vi "BuildZLUT.vi"(11 "MeasureConfig":T2={"Bead locations"=[{"X"=0, "Y"=0}], "ROI"=200, "Experiment base path"=path "", "Image output subdir"="images", "Output mode"=enum."None", "Traces output subdir"="traces", "QTrk Settings"={"Image width"=150, "Image height"=150, "Number of threads (CPU based)"=-1, "CUDA Device"=-2, "COM Background correction factor"=0.0, "ZLUT MinRadius"=8.0, "ZLUT Radial sample density"=5.0, "ZLUT Angular sample density"=2.0, "ZLUT ROI Coverage"=0.7, "QI Iterations"=1, "QI MinRadius"=2.0, "QI Radial sample density"=5.0, "QI Angular sample density"=2.0, "QI ROI Coverage"=0.7, "QI Angular Step \nIteration Factor"=0.8, "XCOR Profile Length"=1, "XCOR Profile Width"=128, "XCOR Iterations"=32, "Gaussian 2D Fit Iterations"=2, "Gaussian 2D Sigma (pixels)"=3.0, "Downsample"=0}, "Tracking Config"={"Number of steps"=0, "ZLUT stepsize (um)"=0.0, "Z correction factor"=0.0, "Start piezo Z (um)"=0.0, "Pixel size (nm)"=0.0, "2D Localization Type"=enum."Quadrant Interpolation", "Z Command (None)"=enum."Nothing", "Z Piezo scale"=FALSE}, "Experiment Name"="", "Program"={"Commands"=[], "Motor Axis accuracy conditions"={"Magnet Z"=0.0, "Magnet rotation"=0.0, "Camera"={"X"=0.0, "Y"=0.0}, "Piezo XY"={"X"=0.0, "Y"=0.0}, "Piezo Z"=0.0}, "Axis flags"={"Magnet Z"=FALSE, "Magnet rotation"=FALSE, "Camera"={"X"=FALSE, "Y"=FALSE}, "Piezo XY"={"X"=FALSE, "Y"=FALSE}, "Piezo Z"=FALSE}}, "ZLUT"=[], "Camera settings"={"Framerate (Hz)"=60, "Exposure time (us)"=5000, "Image size"={"Width"=1280, "Height"=1024}, "Number of buffers"=30}, "Experiment Script"="", "Max frames in memory"=10000, "Save traces as binary"=FALSE, "Pixel Calibration Gain Image"="camera_calib_gain.bin", "Pixel Calibration Offset Image"="camera_calib_offset.bin", "Use pixel calibration images"=FALSE, "Internal camera settings"="", "Trace write interval"=100} {"QTrk Settings"."QI ROI Coverage" format="%_2g"; "QTrk Settings"."QI MinRadius" format="%.2f"; "QTrk Settings"."QI Angular sample density" format="%.3f"; "QTrk Settings"."QI Radial sample density" format="%.2f"; "QTrk Settings"."ZLUT Radial sample density" format="%.2f"; "QTrk Settings"."ZLUT MinRadius" format="%.2f"}) -> (2 "Is cancelled?":bool, 3 "ZLUT":sgl[][][](array[numeric]))   [LabVIEW 2011]
uses:
  Typedefs/MeasureConfigType.ctl
  Typedefs/MeasureConfigOutputMode.ctl
  qtrk/QTrkLVBinding/QTrkSettings.ctl
  Typedefs/TrackingConfigType.ctl
  qtrk/QTrkLVBinding/QTrkLocalizationType.ctl
  qtrk/QTrkLVBinding/QTrkZCommandType.ctl
  ExperimentProgram/ExperimentProgramType.ctl
  ExperimentProgram/ExProgCommandType.ctl
  ExperimentProgram/ExProgCommandEnumType.ctl
  Motors/MotorAxisEnum.ctl
  Motors/MotorPosType.ctl
  Typedefs/XYf.ctl
  Motors/MotorPosFlagsType.ctl
  Camera/GenericCameraConfigType.ctl
  <vilib>/vision/Image Controls.llb/IMAQ Image.ctl
  Camera/CIGrabControlMsg.ctl
  Camera/CIGrabControlMsgEnum.ctl
  GlobalVariables.vi
panel:
  in  "Wait frames after motor move":i32=1
  in  "thread id":i32
  in  "Get debug image?":bool
  out "dbg image":sgl[][](graph)
  in  "Grab Framerate (Hz)":i32=20
  out "Image":T1(plugin-control)
  in  "Check for motor position?":bool=TRUE
  in  "Image available?":bool
  in  "stop capturing":bool
  out "total result count":i32
  out "QTrk result count":i32
  out "Piezo Z":sgl
  in  "Cancel":bool
  out "Frame #":i32
  out "last image grabbed":T1
  out "Total # of steps":i32
  out "Step":i32
  # "Building Z lookup table..."
  # "(used for commands with string parameters)"
  # "-2: Use all devices\n-1: Use best device"
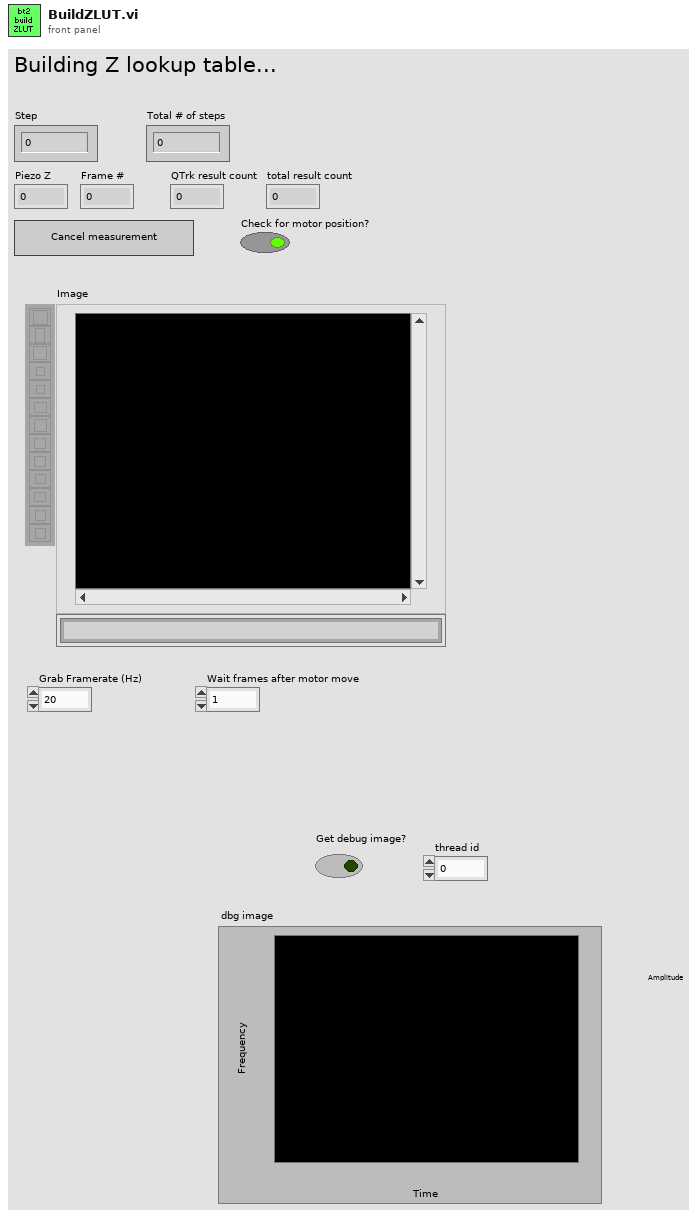
[diagram p1: front panel]
types:
  T1 = typedef "IMAQ Image.ctl" = refnum<image>
  T2 = typedef "MeasureConfigType.ctl" = cluster{"Bead locations":cluster{"X":i32, "Y":i32}[], "ROI":i32, "Experiment base path":path, "Image output subdir":string, "Output mode":T3, "Traces output subdir":string, "QTrk Settings":T4, "Tracking Config":T5, "Experiment Name":string, "Program":T8, "ZLUT":sgl[][][], "Camera settings":T15, "Experiment Script":string, "Max frames in memory":i32, "Save traces as binary":bool, "Pixel Calibration Gain Image":string, "Pixel Calibration Offset Image":string, "Use pixel calibration images":bool, "Internal camera settings":string, "Trace write interval":i32}
  T3 = typedef "MeasureConfigOutputMode.ctl" = enum16{"None", "Track", "SaveImages"}
  T4 = typedef "QTrkSettings.ctl" = cluster{"Image width":i32, "Image height":i32, "Number of threads (CPU based)":i32, "CUDA Device":i32, "COM Background correction factor":sgl, "ZLUT MinRadius":sgl, "ZLUT Radial sample density":sgl, "ZLUT Angular sample density":sgl, "ZLUT ROI Coverage":sgl, "QI Iterations":i32, "QI MinRadius":sgl, "QI Radial sample density":sgl, "QI Angular sample density":sgl, "QI ROI Coverage":sgl, "QI Angular Step \nIteration Factor":sgl, "XCOR Profile Length":i32, "XCOR Profile Width":i32, "XCOR Iterations":i32, "Gaussian 2D Fit Iterations":i32, "Gaussian 2D Sigma (pixels)":sgl, "Downsample":i32}
  T5 = typedef "TrackingConfigType.ctl" = cluster{"Number of steps":i32, "ZLUT stepsize (um)":sgl, "Z correction factor":sgl, "Start piezo Z (um)":sgl, "Pixel size (nm)":sgl, "2D Localization Type":T6, "Z Command (None)":T7, "Z Piezo scale":bool}
  T6 = typedef "QTrkLocalizationType.ctl" = enum16{"Center-of-Mass", "1D Cross-Correlation", "Quadrant Interpolation", "Gaussian 2D MLE", "QI + ZLUTAlign", "ZLUTAlign", "QI + FourierLUT"}
  T7 = typedef "QTrkZCommandType.ctl" = enum16{"Nothing", "ComputeZ", "BuildRadialZLUT", "BuildImageZLUT", "RadialZLUT+ImageZLUT"}
  T8 = typedef "ExperimentProgramType.ctl" = cluster{"Commands":T9[], "Motor Axis accuracy conditions":T12, "Axis flags":T14}
  T9 = typedef "ExProgCommandType.ctl" = cluster{"cmd":T10, "axis":T11, "value/pos":dbl, "speed":dbl, "name":string}
  T10 = typedef "ExProgCommandEnumType.ctl" = enum16{"wait", "move", "acquire", "idle", "rmove", "when", "section", "stop"}
  T11 = typedef "MotorAxisEnum.ctl" = enum16{"no axis", "magrot", "magpos", "px", "py", "pz", "camx", "camy"}
  T12 = typedef "MotorPosType.ctl" = cluster{"Magnet Z":dbl, "Magnet rotation":dbl, "Camera":T13, "Piezo XY":T13, "Piezo Z":dbl}
  T13 = typedef "XYf.ctl" = cluster{"X":sgl, "Y":sgl}
  T14 = typedef "MotorPosFlagsType.ctl" = cluster{"Magnet Z":bool, "Magnet rotation":bool, "Camera":cluster{"X":bool, "Y":bool}, "Piezo XY":cluster{"X":bool, "Y":bool}, "Piezo Z":bool}
  T15 = typedef "GenericCameraConfigType.ctl" = cluster{"Framerate (Hz)":i32, "Exposure time (us)":i32, "Image size":cluster{"Width":i32, "Height":i32}, "Number of buffers":i32}
  T16 = typedef "MotorStateType.ctl" = cluster{"Enabled?":bool, "Current Position":T12, "Update counter":i32}
  T17 = typedef "QTrkInstance.ctl" = cluster{"QTrk Pointer":u64}
  T18 = typedef "QTrkComputedSettings.ctl" = cluster{"QTrk Settings":T4, "Derived settings":cluster{"ZLUT Radial Steps":i32, "ZLUT Angular Steps":i32, "ZLUT Max Radius":sgl, "QI Radial Steps":i32, "QI Angular Steps\nPer Quadrant":i32, "QI Max Radius":sgl}}
  T19 = typedef "CIGrabType.ctl" = refnum<vi>
  T20 = typedef "CmdData_NewFrame.ctl" = cluster{"Buffer Image":T1, "Frame #":i32, "Hardware ROI Index":i32, "Timestamp":dbl, "Type":T21}
  T21 = typedef "CmdEnum_CameraFrameType.ctl" = enum16{"Full", "HardwareROI", "EndGrabMarker"}
  T22 = typedef "CIGrabControlMsg.ctl" = cluster{"Msg":T23}
  T23 = typedef "CIGrabControlMsgEnum.ctl" = enum16{"Stop", "EnableTracking", "DisableTracking"}
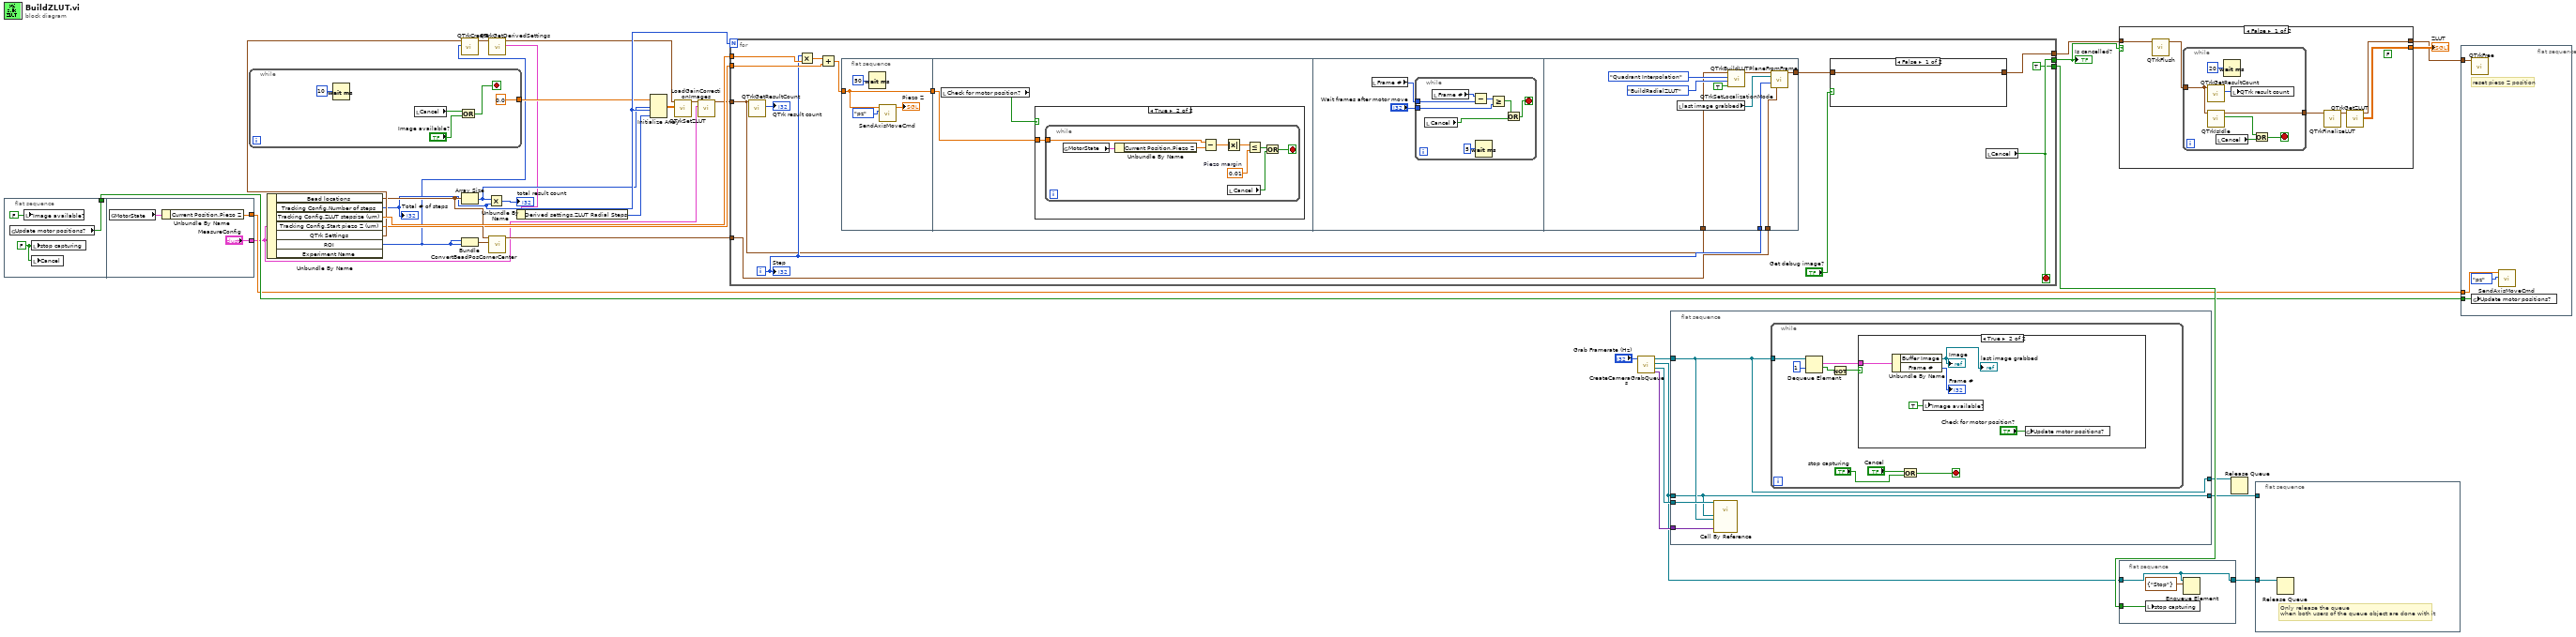
[diagram p0: block diagram]
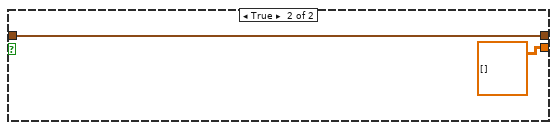
[diagram p3: hidden frame]
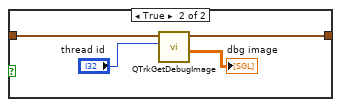
[diagram p4: hidden frame]
diagram:
  n1 = flat-sequence {
    tunnel: [w35] -> w17
    tunnel: ["MeasureConfig"] -> w12
    tunnel: [w38] -> w16
    frame #0 {
      w36 = FALSE ("Cancel")
      n2 = global read "GlobalVariables.vi" "Update motor positions?"() -> (w35:bool)
      n3 = local write "Image available?"(FALSE ("Image available?")) -> ()
      n4 = local write "stop capturing"(w36) -> ()
      n5 = local write "Cancel"(w36) -> ()
    }
    frame #1 {
      n6 = global read "GlobalVariables.vi" "MotorState"() -> (w39:T16)
      n7 = Unbundle By Name(w39) -> ("Current Position.Piezo Z"=w38:dbl)
    }
  }
  n8 = while {
    tunnel: [sgl 0.0 ("element")] -> w22
    stop <- w41 stop-if-true
    n9 = Wait (ms)(milliseconds to wait=u32 10) -> ()  [unwired: 1 out]
    n10 = local read "Cancel"() -> (w43:bool)
    n11 = Or(x=w43, y="Image available?") -> (x .or. y?=w41:bool)
  }
  n12 = Unbundle By Name(w12) -> ("Bead locations"=w31:cluster{"X":i32, "Y":i32}[], "Tracking Config.Number of steps"=w25:i32, "Tracking Config.ZLUT stepsize (um)"=w34:sgl, "Tracking Config.Start piezo Z (um)"=w21:sgl, "QTrk Settings"=w33:T4, "ROI"=w19:i32)  [unwired: 1 out]
  "Total # of steps" <- w25
  n13 = call "QTrkCreate.vi"("ROI"=w19, "QTrk Settings"=w33) -> ("QTrk Instance"=w15:T17)  [unwired: 3 in, 2 out]
  n14 = Array Size(array=w31) -> (size(s)=w20:i32)
  n15 = Bundle("ROI"=w19, "ROI"=w19) -> (w18:cluster{"ROI":i32, "ROI":i32})  [unwired: 1 in]
  n16 = Multiply(x=w20, y=w25) -> (x*y=→"total result count":i32)
  n17 = call "QTrkGetDerivedSettings.vi"("QTrk Instance"=w15) -> ("Derived settings"=w14:T18, "QTrk Instance (out)"=w1:T17)  [unwired: 5 in, 4 out]
  n18 = call "ConvertBeadPosCornerCenter.vi"("ROI Size"=w18, "Center-based bead locations"=w31) -> ("Corner-based bead pos (out)"=w30:cluster{"X":i32, "Y":i32}[])  [unwired: 8 in, 1 out]
  n19 = Unbundle By Name(w14) -> ("Derived settings.ZLUT Radial Steps"=w13:i32)
  n20 = Initialize Array(w22, w20, w25, w13) -> (w32:sgl[][][])
  n21 = call "QTrkSetZLUT.vi"("ZLUT"=w32, "QTrk Instance"=w1) -> ("QTrk Instance"=w11:T17)  [unwired: 8 in, 1 out]
  n22 = call "LoadGainCorrectionImages.vi"("MeasureConfig"=w12, "QTrk Instance in"=w11) -> ("QTrk Instance out"=w10:T17)  [unwired: 9 in]
  n23 = for {
    N: w25 -> [_]
    tunnel: w34 -> [w59]
    tunnel: w21 -> [w57]
    tunnel: w10 -> [w52]
    tunnel: [w46] -> w27
    tunnel: w30 -> [w54]
    tunnel: [w53] -> w26
    tunnel: [TRUE ("stop capturing")] -> w23
    i -> [w55]
    stop <- w53 stop-if-true
    n24 = call "QTrkGetResultCount.vi"("QTrk Instance"=w52) -> ("result count"=→"QTrk result count":i32)  [unwired: 4 in, 2 out]
    n25 = Multiply(x=w55, y=w59) -> (x*y=w58:sgl)
    n26 = Add(x=w58, y=w57) -> (x+y=w56:sgl)
    n27 = flat-sequence {
      tunnel: w56 -> [w67]
      tunnel: [w67] -> w49
      tunnel: w49 -> [w70]
      tunnel: w52 -> [w96]
      tunnel: w55 -> [w94]
      tunnel: [w92] -> w47
      tunnel: w54 -> [w93]
      frame #0 {
        n28 = Wait (ms)(milliseconds to wait=u32 50) -> ()  [unwired: 1 out]
        n29 = call "SendAxisMoveCmd.vi"("axis"=MotorAxisEnum."pz", "Position"=w67) -> ("Limited pos"=→"Piezo Z":dbl)  [unwired: 9 in]
      }
      frame #1 {
        n30 = local read "Check for motor position?"() -> (w69:bool)
        n31 = case shown="True" w69 {
          tunnel: w70 -> [_ w71]
          frame False {
          }
          frame True {
            n32 = while {
              tunnel: w71 -> [w77]
              stop <- w78 stop-if-true
              w73 = 0.01  # Piezo margin
              n33 = global read "GlobalVariables.vi" "MotorState"() -> (w80:T16)
              n34 = Unbundle By Name(w80) -> ("Current Position.Piezo Z"=w76:dbl)
              n35 = Subtract(x=w77, y=w76) -> (x-y=w75:dbl)
              n36 = Absolute Value(x=w75) -> (abs(x)=w74:dbl)
              n37 = local read "Cancel"() -> (w79:bool)
              n38 = Less Or Equal?(x=w74, y=w73) -> (x <= y?=w72:bool)
              n39 = Or(x=w72, y=w79) -> (x .or. y?=w78:bool)
            }
          }
        }
      }
      frame #2 {
        n40 = local read "Frame #"() -> (w82:i32)
        n41 = while {
          tunnel: w82 -> [w89]
          tunnel: "Wait frames after motor move" -> [w87]
          stop <- w84 stop-if-true
          n42 = local read "Cancel"() -> (w83:bool)
          n43 = local read "Frame #"() -> (w90:i32)
          n44 = Subtract(x=w90, y=w89) -> (x-y=w88:i32)
          n45 = Wait (ms)(milliseconds to wait=u32 5) -> ()  [unwired: 1 out]
          n46 = Greater Or Equal?(x=w88, y=w87) -> (x >= y?=w85:bool)
          n47 = Or(x=w85, y=w83) -> (x .or. y?=w84:bool)
        }
      }
      frame #3 {
        n48 = local read "last image grabbed"() -> (w91:T1)
        n49 = call "QTrkSetLocalizationMode.vi"("Normalize profile"=TRUE, "Z Command"=QTrkZCommandType."BuildRadialZLUT", "2D Localization Type"=QTrkLocalizationType."Quadrant Interpolation", "QTrk Instance"=w96) -> ("QTrk Instance"=w95:T17)  [unwired: 7 in]
        n50 = call "QTrkBuildLUTPlaneFromFrame.vi"("QTrk Instance"=w95, "Image"=w91, "plane"=w94, "ROI Positions (corner-based)"=w93) -> ("QTrk Instance"=w92:T17)  [unwired: 11 in]
      }
    }
    n51 = case shown="False" "Get debug image?" {
      tunnel: w47 -> [w60 w64]
      tunnel: [w60 w63] -> w46
      frame False {
      }
      frame True {
        n52 = call "QTrkGetDebugImage.vi"("id"="thread id", "QTrk Instance"=w64) -> ("data"=→"dbg image":sgl[][], "QTrk Instance (out)"=w63:T17)  [unwired: 7 in, 1 out]
      }
    }
    n53 = local read "Cancel"() -> (w53:bool)
    "Step" <- w55
  }
  "Is cancelled?" <- w26
  n54 = call "CreateCameraGrabQueues.vi"("Framerate (Hz)"="Grab Framerate (Hz)") -> ("Camera state (out)"=w7:variant, "VI refs.Grab"=w8:T19, "GrabControlQueue"=w4:refnum<queue>, "CameraOutQueue"=w6:refnum<queue>)  [unwired: 7 in]
  n55 = flat-sequence {
    tunnel: w8 -> [w103]
    tunnel: w7 -> [w102]
    tunnel: w6 -> [w101]
    tunnel: w4 -> [w100]
    tunnel: [w101] -> w5
    tunnel: [w100] -> w2
    frame #0 {
      n56 = call-by-ref "?"(reference=w103, "Camera data"=w102, "Output Queue"=w101, "GrabControlQueue"=w100) -> ()  [unwired: 9 in, 3 out]
      n57 = while {
        tunnel: w101 -> [w104]
        stop <- w109 stop-if-true
        n58 = Dequeue Element(queue=w104, timeout in ms (-1)=1) -> (element=w107:T20, timed out?=w106:bool)  [unwired: 1 in, 2 out]
        n59 = Not(x=w106) -> (.not. x?=w105:bool)
        n60 = case shown="True" w105 {
          tunnel: w107 -> [_ w116]
          frame False {
          }
          frame True {
            n61 = Unbundle By Name(w116) -> ("Buffer Image"=→"last image grabbed" →"Image":T1, "Frame #"=→"Frame #":i32)
            n62 = local write "Image available?"(TRUE ("Image available?")) -> ()
            n63 = global write "GlobalVariables.vi" "Update motor positions?"("Check for motor position?") -> ()
          }
        }
        n64 = Or(x="Cancel", y="stop capturing") -> (x .or. y?=w109:bool)
      }
    }
  }
  n65 = case shown="False" w26 {
    tunnel: [w122 sgl[][][] [] ("zlut")] -> w29
    tunnel: [w119 w131] -> w28
    tunnel: w27 -> [w121 w131]
    frame False {
      (unwired) FALSE ("Send UI update event? (T)")
      n66 = call "QTrkFlush.vi"("QTrk Instance"=w121) -> ("QTrk Instance (out)"=w120:T17)  [unwired: 9 in, 1 out]
      n67 = while {
        tunnel: w120 -> [w127]
        tunnel: [w129] -> w118
        stop <- w123 stop-if-true
        n68 = call "QTrkGetResultCount.vi"("QTrk Instance"=w127) -> ("result count"=w126:i32)  [unwired: 4 in, 2 out]
        n69 = call "QTrkIsIdle.vi"("QTrk Instance"=w127) -> ("Currently idle?"=w124:bool, "QTrk Instance (out)"=w129:T17)  [unwired: 8 in, 1 out]
        n70 = local read "Cancel"() -> (w125:bool)
        n71 = Wait (ms)(milliseconds to wait=u32 20) -> ()  [unwired: 1 out]
        n72 = local write "QTrk result count"(w126) -> ()
        n73 = Or(x=w124, y=w125) -> (x .or. y?=w123:bool)
      }
      n74 = call "QTrkFinalizeLUT.vi"("QTrk Instance"=w118) -> ("QTrk Instance"=w117:T17)  [unwired: 5 in, 1 out]
      n75 = call "QTrkGetZLUT.vi"("QTrk Instance (in)"=w117) -> ("zlut"=w122:sgl[][][], "QTrk Instance"=w119:T17)  [unwired: 8 in, 1 out]
    }
    frame True {
    }
  }
  "ZLUT" <- w29
  n76 = flat-sequence {
    tunnel: w23 -> [w134]
    tunnel: w4 -> [w132]
    tunnel: [w132] -> w3
    frame #0 {
      n77 = local write "stop capturing"(w134) -> ()
      n78 = Enqueue Element(queue=w132, element=T22 {"Msg"=enum."Stop"}) -> ()  [unwired: 2 in, 3 out]
    }
  }
  n79 = Release Queue(queue=w5) -> ()  [unwired: 2 in, 3 out]
  n80 = flat-sequence {
    tunnel: w3 -> [w135]
    tunnel: w2 -> [_]
    frame #0 {
      # "Only release the queue\nwhen both users of the queue object are done with it"
      n81 = Release Queue(queue=w135) -> ()  [unwired: 2 in, 3 out]
    }
  }
  n82 = flat-sequence {
    tunnel: w28 -> [w139]
    tunnel: w16 -> [w137]
    tunnel: w17 -> [w138]
    frame #0 {
      # "reset piezo Z position"
      n83 = call "QTrkFree.vi"("QTrk Instance"=w139) -> ()  [unwired: 6 in, 1 out]
      n84 = global write "GlobalVariables.vi" "Update motor positions?"(w138) -> ()
      n85 = call "SendAxisMoveCmd.vi"("axis"=MotorAxisEnum."pz", "Position"=w137) -> ()  [unwired: 9 in, 1 out]
    }
  }
